vi "seleccionar offset.vi"() -> ()   [LabVIEW 2015]
uses:
  variables offset.vi
panel:
  in  "stop":bool
  out "valor 7":dbl
  out "valor 6":dbl
  out "valor 5":dbl
  in  "carga":bool
  in  "presion":bool
  in  "lvdt":bool
  # "Offset"
  # "Sensor"
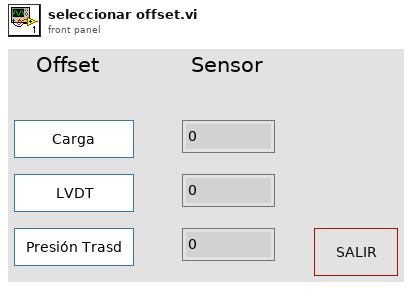
[diagram p1: front panel]
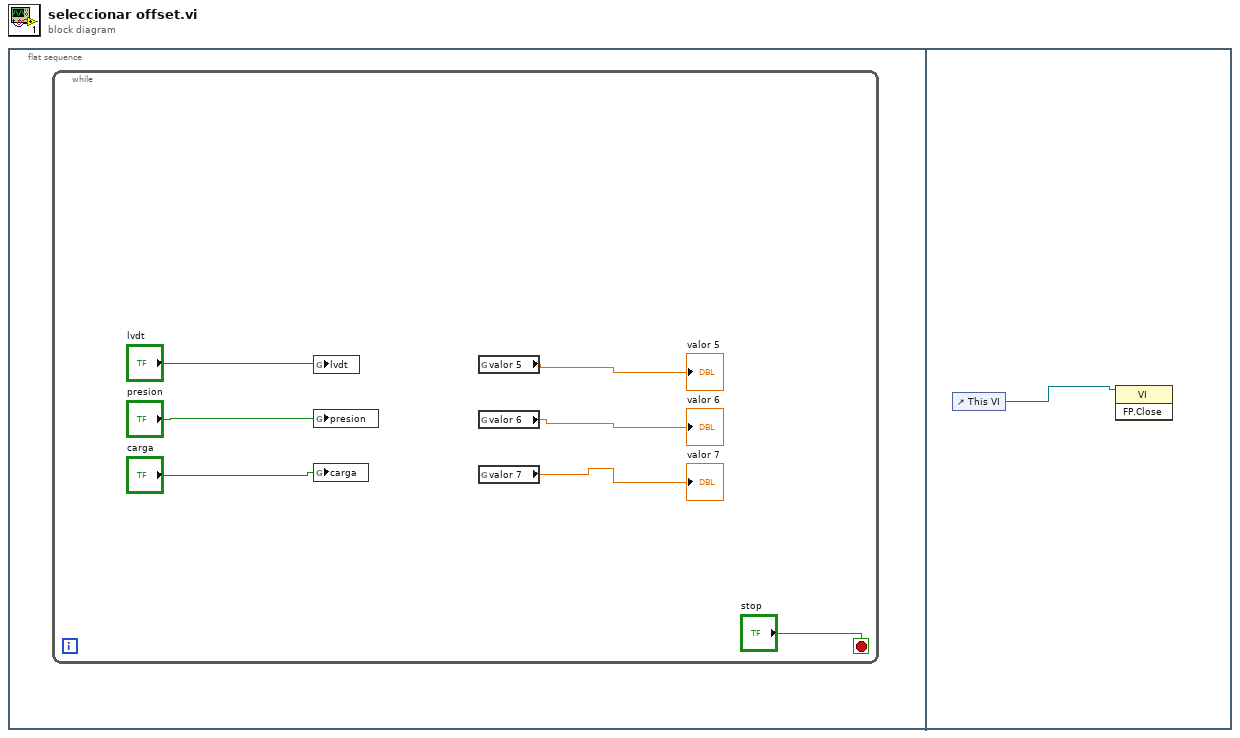
[diagram p0: block diagram]
diagram:
  n1 = flat-sequence {
    frame #0 {
      n2 = while {
        stop <- "stop" stop-if-true
        n3 = global write "variables offset.vi" "lvdt"("lvdt") -> ()
        n4 = global write "variables offset.vi" "presion"("presion") -> ()
        n5 = global write "variables offset.vi" "carga"("carga") -> ()
        n6 = global read "variables offset.vi" "valor 5"() -> (→"valor 5":dbl)
        n7 = global read "variables offset.vi" "valor 6"() -> (→"valor 6":dbl)
        n8 = global read "variables offset.vi" "valor 7"() -> (→"valor 7":dbl)
      }
    }
    frame #1 {
      n9 = control-ref of="This VI"() -> (w8:refnum<vi>)
      n10 = invoke class="VI" method="FP.Close"(reference=w8) -> ()  [unwired: 2 in, 3 out]
    }
  }
